vi "Generate Error.vi"(7 "Is Warning? (False)":bool, 8 "Error In":errorcluster, 9 "Arguments":string[](array[string]), 10 "Error Type":T5, 11 "LINX Device Config":T1) -> (0 "Error Out":errorcluster, 3 "Dup LINX Device Config":T1)   [LabVIEW 2020, in "LMH-LINX.lvlib"]
doc: "Generate a LINX error based on the Error Type input."
uses:
  LMH-LINX.lvlib
  Type Defs/Error Type.ctl
  Device/Type Defs/LINX Device Config.ctl
  Type Defs/Interface.ctl
  Device/Type Defs/TCP Config.ctl
  Device/Type Defs/Channels.ctl
  Device/Device.lvlib
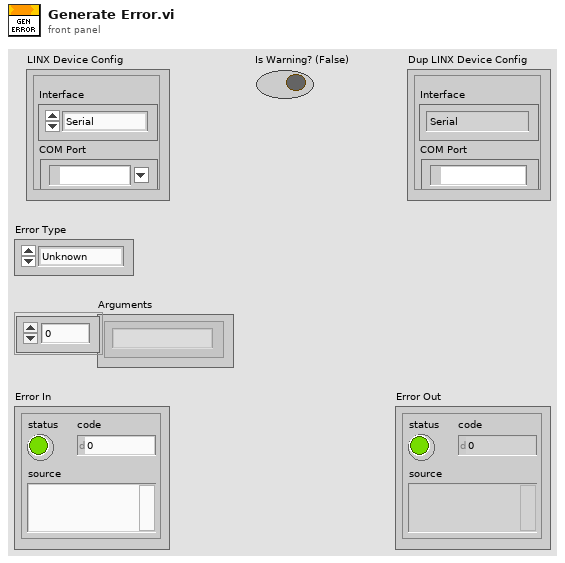
[diagram p1: front panel]
types:
  T1 = typedef "LMH-LINX.lvlib/Device.lvlib/LINX Device Config.ctl" = cluster{"Interface":T2, "COM Port":refnum<visa-resource-name>, "TCP Configuration":T3, "Device Family":u8, "Device ID":u8, "Device Name":string, "TCP Ref":refnum<k5>, "Channels":T4}
  T2 = typedef "LMH-LINX.lvlib/Interface.ctl" = enum16{"Serial", "TCP"}
  T3 = typedef "LMH-LINX.lvlib/Device.lvlib/TCP Config.ctl" = cluster{"IP Address":string, "Port":u16}
  T4 = typedef "LMH-LINX.lvlib/Channels.ctl" = cluster{"DI":u8[], "DO":u8[], "AI":u8[], "AO":u8[], "PWM":u8[], "QE":u8[], "UART":u8[], "I2C 2":u8[], "SPI":u8[], "CAN":u8[], "Servo":u8[], "AI Ref (V)":dbl, "AI Resolution (Bits)":u8, "AO Ref (V)":dbl, "AO Resolution (Bits)":u8}
  T5 = typedef "LMH-LINX.lvlib/Error Type.ctl" = enum16{"Unknown", "Timeout", "Corrupt Return Packet", "Unable To Connect", "Command Not Supported", "Channel DNE", "Invalid COM Config", "Firmware Version Mismatch", "myRIO Support", "CMD Specific Error", "Local IO Not Supported"}
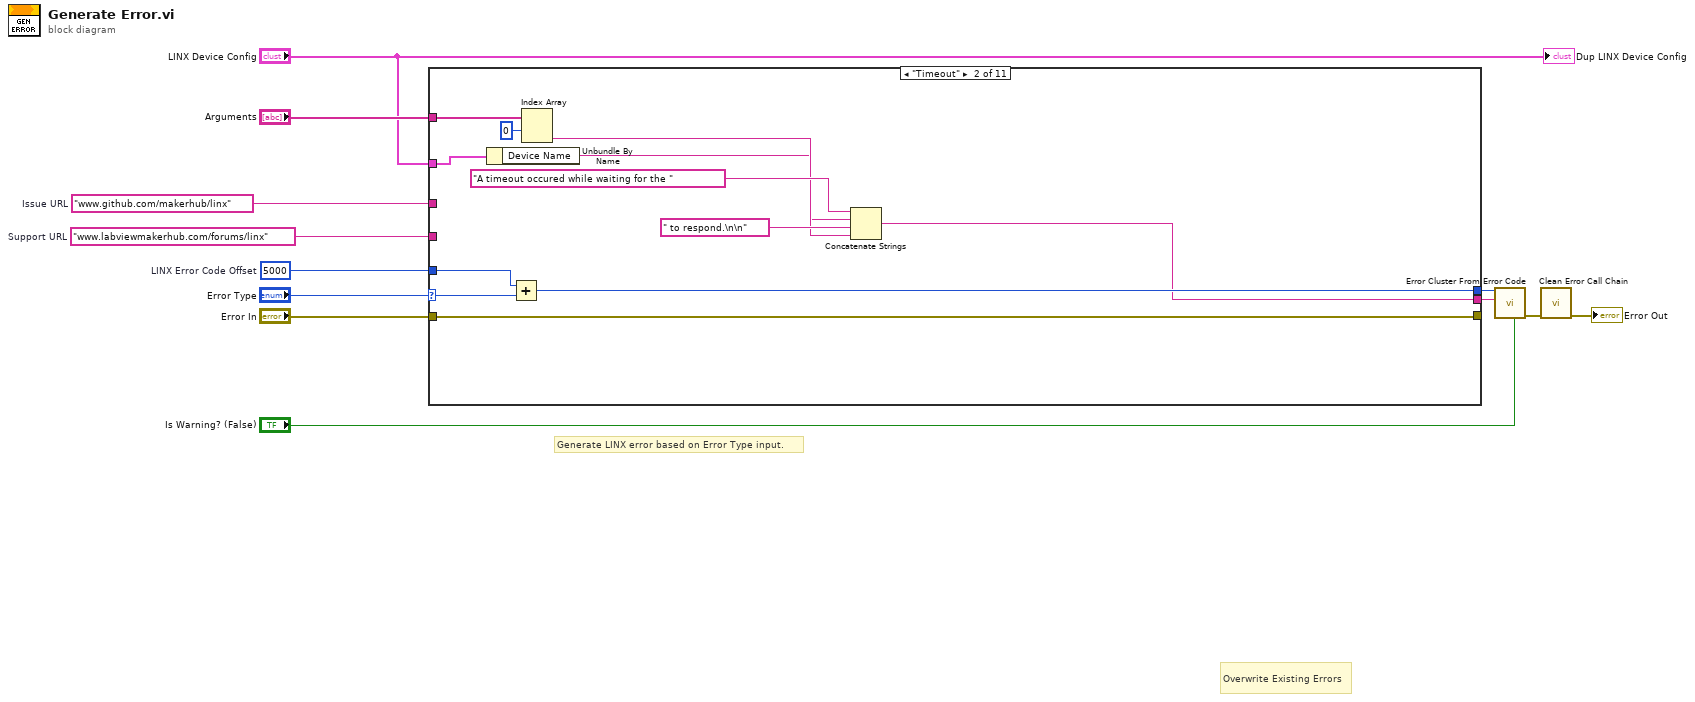
[diagram p0: block diagram]
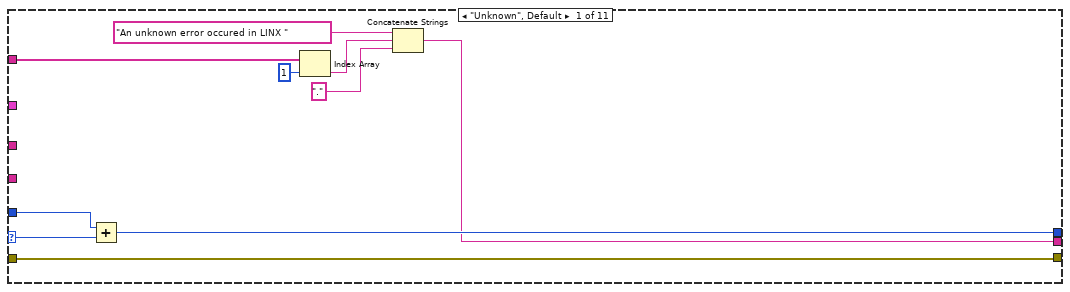
[diagram p2: hidden frame]
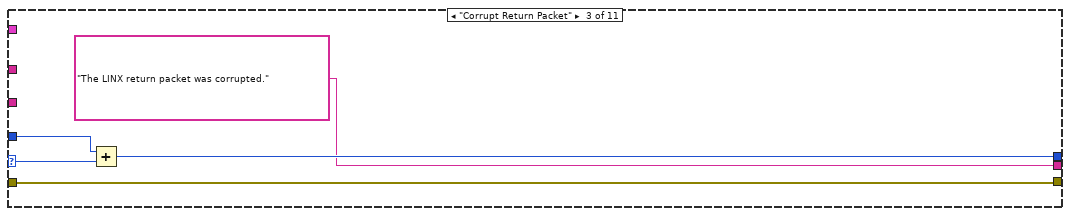
[diagram p3: hidden frame]
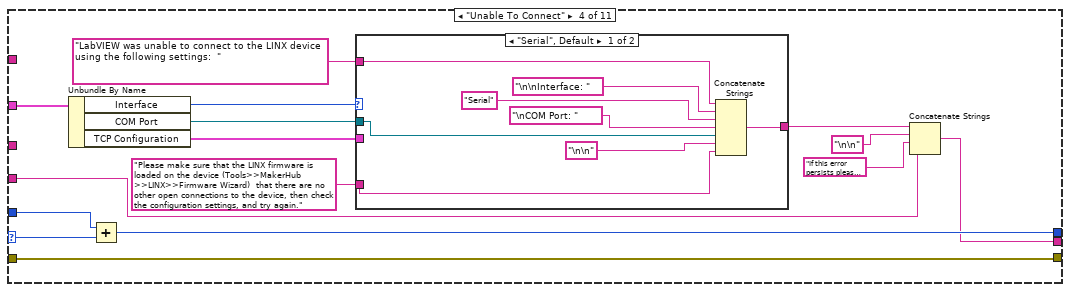
[diagram p4: hidden frame]
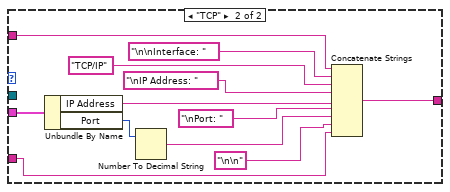
[diagram p5: hidden frame]
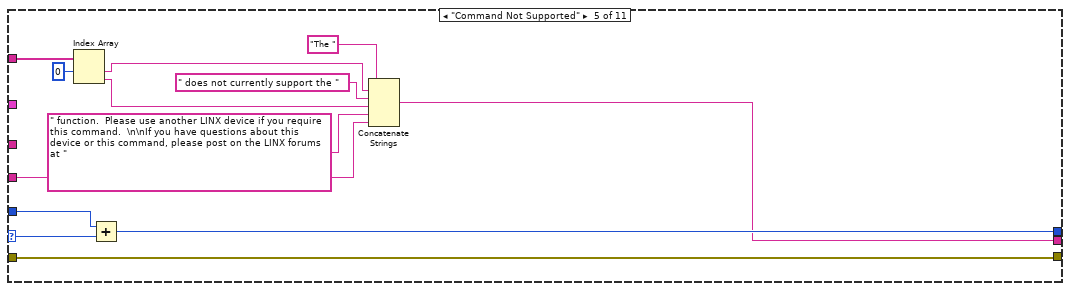
[diagram p6: hidden frame]
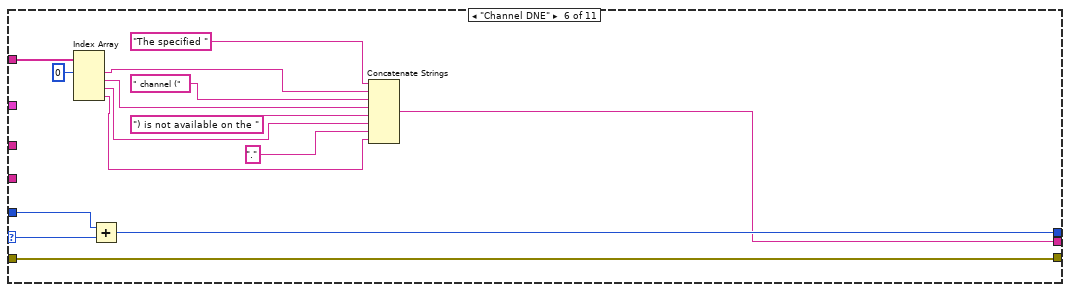
[diagram p7: hidden frame]
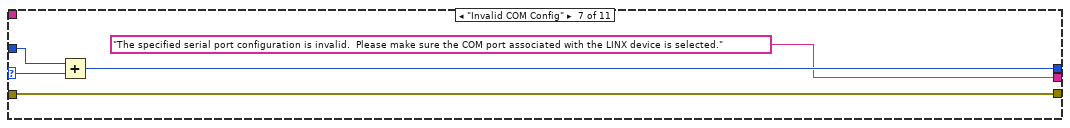
[diagram p8: hidden frame]
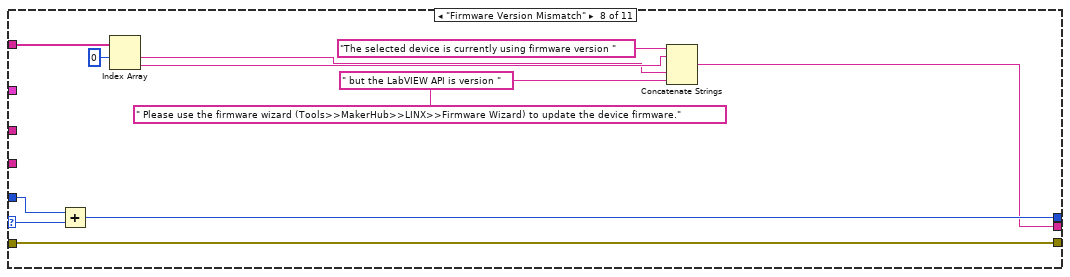
[diagram p9: hidden frame]
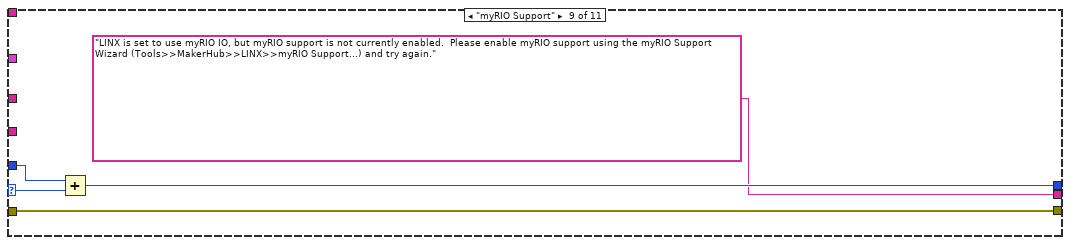
[diagram p10: hidden frame]
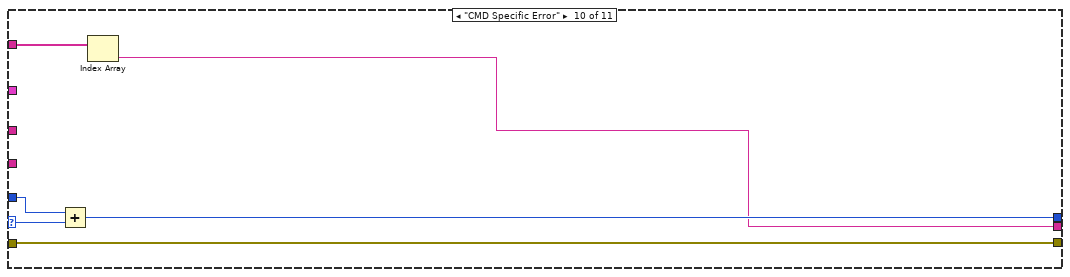
[diagram p11: hidden frame]
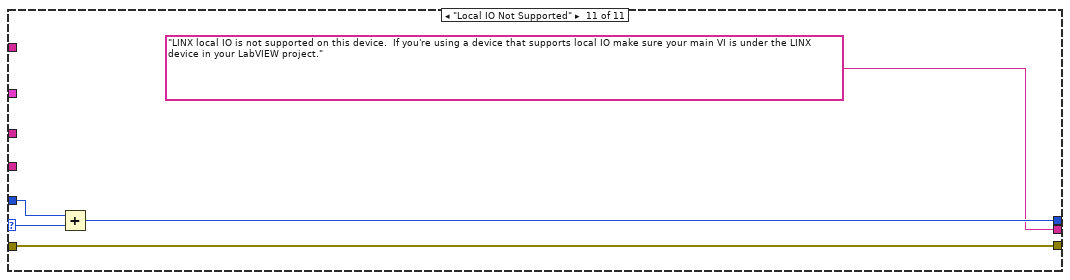
[diagram p12: hidden frame]
diagram:
  w3 = "www.labviewmakerhub.com/forums/linx"  # Support URL
  w6 = "www.github.com/makerhub/linx"  # Issue URL
  w11 = 5000  # LINX Error Code Offset
  # "Overwrite Existing Errors"
  # "Generate LINX error based on Error Type input."
  n1 = case shown="\"Timeout\"" "Error Type" {
    selector: "Error Type" -> [w21 w33 w38 w53 w86 w101 w106 w118 w123 w129 w134]
    tunnel: "Error In" -> [w20 w31 w35 w52 w85 w100 w103 w116 w121 w127 w132]
    tunnel: [w20 w31 w35 w52 w85 w100 w103 w116 w121 w127 w132] -> _
    tunnel: w11 -> [w22 w34 w39 w54 w87 w102 w107 w119 w124 w130 w135]
    tunnel: [w14 w29 "The LINX return packet was corrupted." ("error message (\"\")") w41 w81 w98 "The specified serial port configuration is invalid.  Please make sure the COM port associated with the LINX device is selected." w108 "LINX is set to use myRIO IO, but myRIO support is not currently enabled.  Please enable myRIO support using the myRIO Support Wizard (Tools>>MakerHub>>LINX>>myRIO Support...) and try again." ("Issue URL") w125 "LINX local IO is not supported on this device.  If you're using a device that supports local IO make sure your main VI is under the LINX device in your LabVIEW project." ("Arguments")] -> w9
    tunnel: [w19 w32 w37 w51 w84 w99 w105 w117 w122 w128 w133] -> w8
    tunnel: w6 -> [_ _ _ _ _ _ _ _ _ _ _]
    tunnel: "Arguments" -> [w17 w28 _ _ w79 w97 _ w115 _ w126 _]
    tunnel: "LINX Device Config" -> [_ w24 _ w50 _ _ _ _ _ _ _]
    tunnel: w3 -> [_ _ _ w40 w76 _ _ _ _ _ _]
    frame "Unknown", Default {
      n2 = Add(x=w22, y=w21) -> (x+y=w19:i32)
      n3 = Index Array(array=w17, index=1) -> (element=w16:string)
      n4 = Concatenate Strings("An unknown error occured in LINX " ("error message (\"\")"), w16, "." ("string")) -> (w14:string)
    }
    frame "Timeout" {
      n5 = Unbundle By Name(w24) -> ("Device Name"=w23:string)
      n6 = Add(x=w34, y=w33) -> (x+y=w32:i32)
      n7 = Index Array(array=w28, index #1=0 ("index")) -> (element #2=w25:string)  [unwired: 1 in, 1 out]
      n8 = Concatenate Strings("A timeout occured while waiting for the " ("error message (\"\")"), w23, " to respond.\n\n" ("string"), w25) -> (w29:string)
    }
    frame "Corrupt Return Packet" {
      n9 = Add(x=w39, y=w38) -> (x+y=w37:i32)
    }
    frame "Unable To Connect" {
      n10 = Unbundle By Name(w50) -> ("Interface"=w49:T2, "COM Port"=w45:refnum<visa-resource-name>, "TCP Configuration"=w48:T3)
      n11 = Add(x=w54, y=w53) -> (x+y=w51:i32)
      n12 = case shown="\"Serial\", Default" w49 {
        tunnel: w48 -> [_ w74]
        tunnel: "LabVIEW was unable to connect to the LINX device using the following settings:  " ("error message (\"\")") -> [w59 w70]
        tunnel: "Please make sure that the LINX firmware is loaded on the device (Tools>>MakerHub >>LINX>>Firmware Wizard)  that there are no other open connections to the device, then check the configuration settings, and try again." -> [w55 w64]
        tunnel: [w57 w63] -> w44
        tunnel: w45 -> [w58 _]
        frame "Serial", Default {
          n13 = Concatenate Strings(w59, "\n\nInterface: " ("string"), "Serial" ("string"), "\nCOM Port: " ("string"), w58, "\n\n" ("string"), w55) -> (w57:string)
        }
        frame "TCP" {
          n14 = Unbundle By Name(w74) -> ("IP Address"=w68:string, "Port"=w73:u16)
          n15 = Number To Decimal String(number=w73) -> (decimal integer string=w66:string)  [unwired: 1 in]
          n16 = Concatenate Strings(w70, "\n\nInterface: " ("string"), "TCP/IP" ("string"), "\nIP Address: " ("string"), w68, "\nPort: " ("string"), w66, "\n\n" ("string"), w64) -> (w63:string)
        }
      }
      n17 = Concatenate Strings(w44, "\n\n" ("string"), "If this error persists please search, then post on the LINX forums at " ("error message (\"\")"), w40) -> (w41:string)
    }
    frame "Command Not Supported" {
      n18 = Index Array(array=w79, index #1=0 ("index")) -> (element #1=w75:string, element #2=w77:string)  [unwired: 1 in]
      n19 = Add(x=w87, y=w86) -> (x+y=w84:i32)
      n20 = Concatenate Strings("The " ("string"), w75, " does not currently support the " ("string"), w77, " function.  Please use another LINX device if you require this command.  \n\nIf you have questions about this device or this command, please post on the LINX forums at " ("string"), w76) -> (w81:string)
    }
    frame "Channel DNE" {
      n21 = Index Array(array=w97, index #1=0 ("index")) -> (element #1=w95:string, element #2=w94:string, element #3=w90:string, element #4=w88:string)  [unwired: 3 in]
      n22 = Add(x=w102, y=w101) -> (x+y=w99:i32)
      n23 = Concatenate Strings("The specified ", w95, " channel (" ("string"), w94, ") is not available on the " ("string"), w90, "." ("string"), w88) -> (w98:string)
    }
    frame "Invalid COM Config" {
      n24 = Add(x=w107, y=w106) -> (x+y=w105:i32)
    }
    frame "Firmware Version Mismatch" {
      n25 = Add(x=w119, y=w118) -> (x+y=w117:i32)
      n26 = Index Array(array=w115, index #1=0 ("index")) -> (element #1=w110:string, element #2=w112:string)  [unwired: 1 in]
      n27 = Concatenate Strings("The selected device is currently using firmware version " ("Issue URL"), w112, " but the LabVIEW API is version " ("Issue URL"), w110, " Please use the firmware wizard (Tools>>MakerHub>>LINX>>Firmware Wizard) to update the device firmware." ("Issue URL")) -> (w108:string)
    }
    frame "myRIO Support" {
      n28 = Add(x=w124, y=w123) -> (x+y=w122:i32)
    }
    frame "CMD Specific Error" {
      n29 = Add(x=w130, y=w129) -> (x+y=w128:i32)
      n30 = Index Array(array=w126) -> (element=w125:string)  [unwired: 1 in]
    }
    frame "Local IO Not Supported" {
      n31 = Add(x=w135, y=w134) -> (x+y=w133:i32)
    }
  }
  n32 = call <vilib>:"Error Cluster From Error Code.vi"("is warning? (False)"="Is Warning? (False)", "error message (\"\")"=w9, "error code (0)"=w8) -> ("error out"=w2:errorcluster)  [unwired: 6 in]
  n33 = call "Clean Error Call Chain.vi"("Error In"=w2) -> ("Error Out"=→"Error Out":errorcluster)  [unwired: 10 in]
  "Dup LINX Device Config" <- "LINX Device Config"
